vi "Clear_Log.vi"   [LabVIEW 2011]
doc: "This VI clears the global \"Log\" variable."
uses:
  low_level_proc/globals.vi
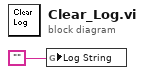
[diagram p0: block diagram]
diagram:
  n1 = global write "globals.vi" "Log String"("") -> ()
